vi "Constants.vi"() -> ()   [LabVIEW 2020, in "AIM ARINC 664 Shared.lvlib"]
doc: "Use this Global VI to access the GUIDs assigned to the page resources of the Custom Device."
uses:
  AIM ARINC 664 Shared.lvlib
panel:
  in  "Tab Control":enum32{"GUIDs", "Constants", "Properties"}(tab)=enum."Constants"
  in  "RTM Wrapper":string="FC841DFB-0C48-4F2C-A4DD-E549408A50F6"
  in  "Compiled.Settings":string="Compiled.Settings"
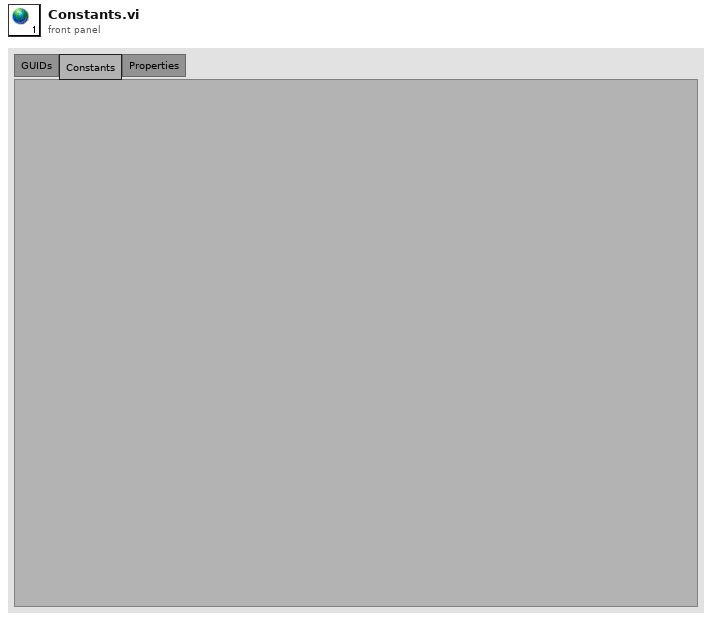
[diagram p1: front panel]
diagram:
